vi "실습2-1숫자형데이터삽입.vi"() -> ()   [LabVIEW 2014]
panel:
  out "sin(x)":dbl format="%#_6f"
  in  "A":dbl
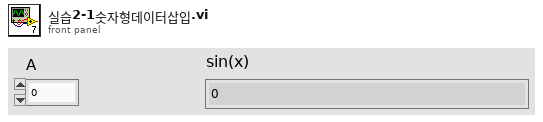
[diagram p1: front panel]
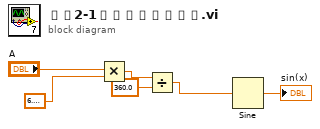
[diagram p0: block diagram]
diagram:
  n1 = Multiply(x="A", y=6.283185307179586) -> (x*y=w6:dbl)
  n2 = Divide(x=w6, y=360.0) -> (x/y=w2:dbl)
  n3 = Sine(x=w2) -> (sin(x)=→"sin(x)":dbl)
